vi "Read Operatator Joystick.vi"(11 "Operator Joystick":T1) -> ()   [LabVIEW 2019]
uses:
  <vilib>/Rock Robotics/WPI/Joystick/WPI_JoystickDevRef.ctl
  <vilib>/Rock Robotics/WPI/Joystick/WPI_JoystickDeviceEnum.ctl
  Controls/Joystick Mini Sticks.ctl
  Controls/Joystick Buttons.ctl
  Framework/Robot Global Data.vi
panel:
  # "READ OPERATOR JOYSTICK"
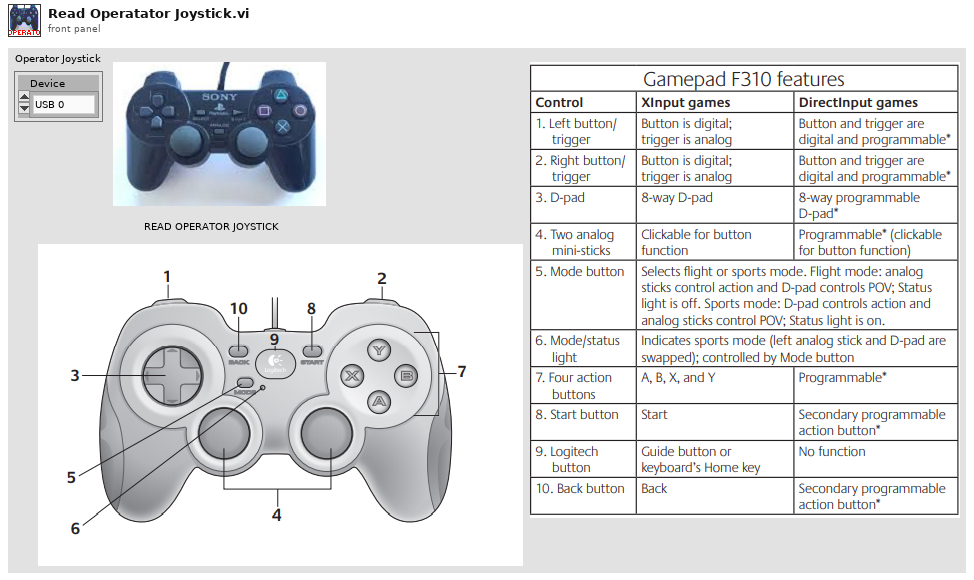
[diagram p1: front panel]
types:
  T1 = typedef "WPI_JoystickDevRef.ctl" = cluster{"Device":T2}
  T2 = typedef "WPI_JoystickDeviceEnum.ctl" = enum16{"USB 0", "USB 1", "USB 2", "USB 3", "USB 4", "USB 5"}
  T3 = typedef "Joystick Buttons.ctl" = enum16{"Triangle 0", "Circle 1", "X 2", "Square 3", "Left Button 4", "Right Button 5", "Left Trigger 6", "Right Trigger 7"}
  T4 = typedef "Joystick Mini Sticks.ctl" = enum16{"Left Stick 0: X Axis", "Left Stick 1: Y Axis", "Right Stick 2: Z Axis", "Right Stick 3: Z Rotates"}
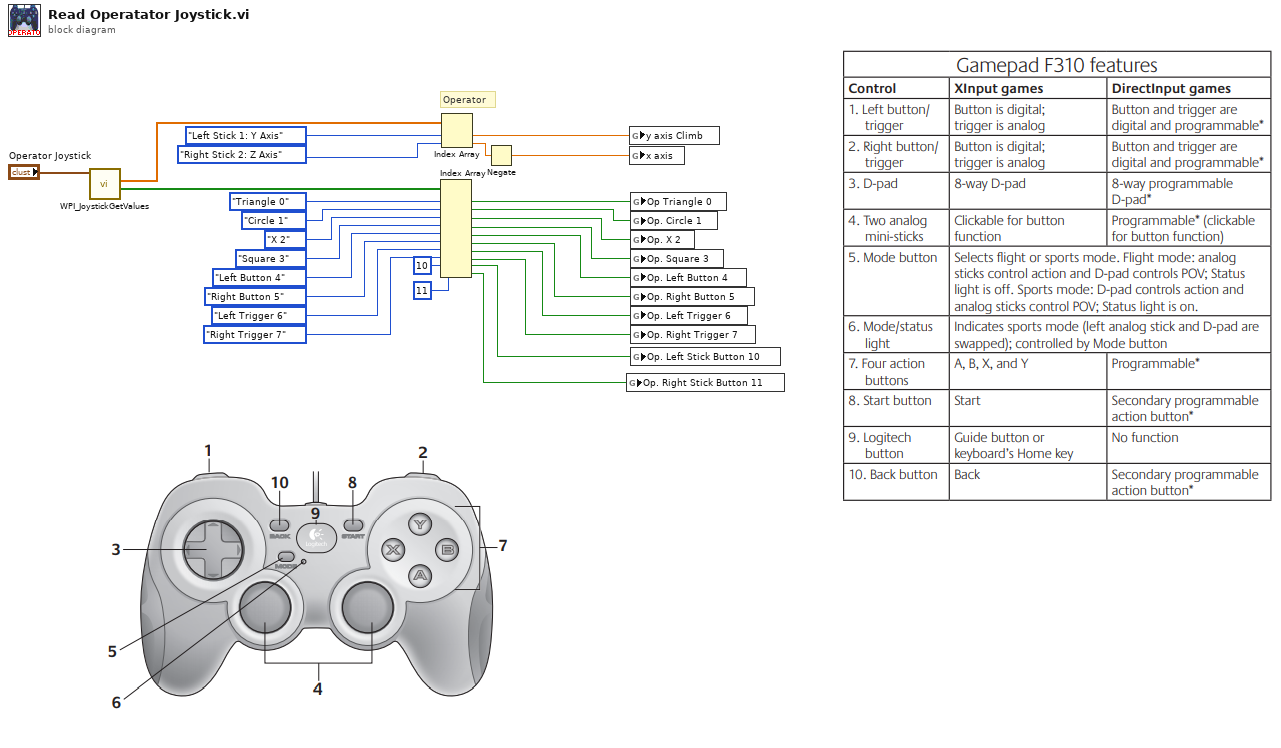
[diagram p0: block diagram]
diagram:
  # "Operator"
  n1 = call <vilib>:"WPI_JoystickGetValues.vi"("JoystickDevRef"="Operator Joystick") -> ("Buttons"=w26:bool[], "Axes"=w25:dbl[])  [unwired: 6 in, 3 out]
  n2 = Index Array(array=w26, index #1=Joystick_Buttons."Triangle 0" ("Joystick Buttons"), index #2=Joystick_Buttons."Circle 1" ("Joystick Buttons"), index #3=Joystick_Buttons."X 2" ("Joystick Buttons"), index #4=Joystick_Buttons."Square 3" ("Joystick Buttons"), index #5=Joystick_Buttons."Left Button 4" ("Joystick Buttons"), index #6=Joystick_Buttons."Right Button 5" ("Joystick Buttons"), index #7=Joystick_Buttons."Left Trigger 6" ("Joystick Buttons"), index #8=Joystick_Buttons."Right Trigger 7" ("Joystick Buttons"), index #9=10 ("index"), index #10=11 ("index")) -> (element #1=w27:bool, element #2=w24:bool, element #3=w23:bool, element #4=w19:bool, element #5=w22:bool, element #6=w21:bool, element #7=w20:bool, element #8=w18:bool, element #9=w3:bool, element #10=w1:bool)
  n3 = Index Array(array=w25, index #1=Joystick_Mini_Sticks."Left Stick 1: Y Axis" ("Joystick Mini Sticks"), index #2=Joystick_Mini_Sticks."Right Stick 2: Z Axis" ("Joystick Mini Sticks")) -> (element #1=w17:dbl, element #2=w28:dbl)
  n4 = Negate(x=w28) -> (-x=w16:dbl)
  n5 = global write "Robot Global Data.vi" "Op. Right Stick Button 11"(w1) -> ()
  n6 = global write "Robot Global Data.vi" "y axis Climb"(w17) -> ()
  n7 = global write "Robot Global Data.vi" "x axis"(w16) -> ()
  n8 = global write "Robot Global Data.vi" "Op Triangle 0"(w27) -> ()
  n9 = global write "Robot Global Data.vi" "Op. Circle 1"(w24) -> ()
  n10 = global write "Robot Global Data.vi" "Op. X 2"(w23) -> ()
  n11 = global write "Robot Global Data.vi" "Op. Square 3"(w19) -> ()
  n12 = global write "Robot Global Data.vi" "Op. Left Button 4"(w22) -> ()
  n13 = global write "Robot Global Data.vi" "Op. Right Button 5"(w21) -> ()
  n14 = global write "Robot Global Data.vi" "Op. Left Trigger 6"(w20) -> ()
  n15 = global write "Robot Global Data.vi" "Op. Right Trigger 7"(w18) -> ()
  n16 = global write "Robot Global Data.vi" "Op. Left Stick Button 10"(w3) -> ()
